vi "DAQNavi Write (Analog 1D Wfm NChan 1Samp).vi"(8 "error in (no error)":errorcluster, 9 "timeout":dbl=10.0, 10 "data":waveform(dbl)[](array[waveform]), 11 "task in":i32) -> (0 "error out":errorcluster, 2 "number of samples written per channel":u32, 3 "task out":i32)   [LabVIEW 2020]
uses:
  DAQNavi_LV.dll
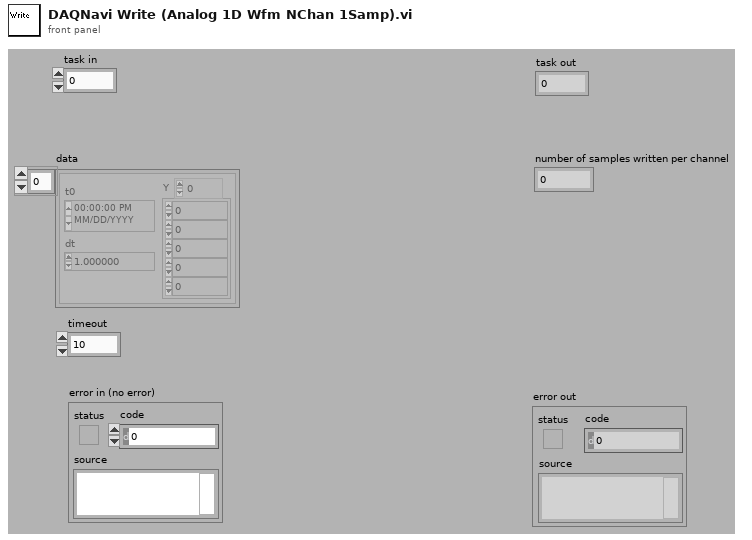
[diagram p1: front panel]
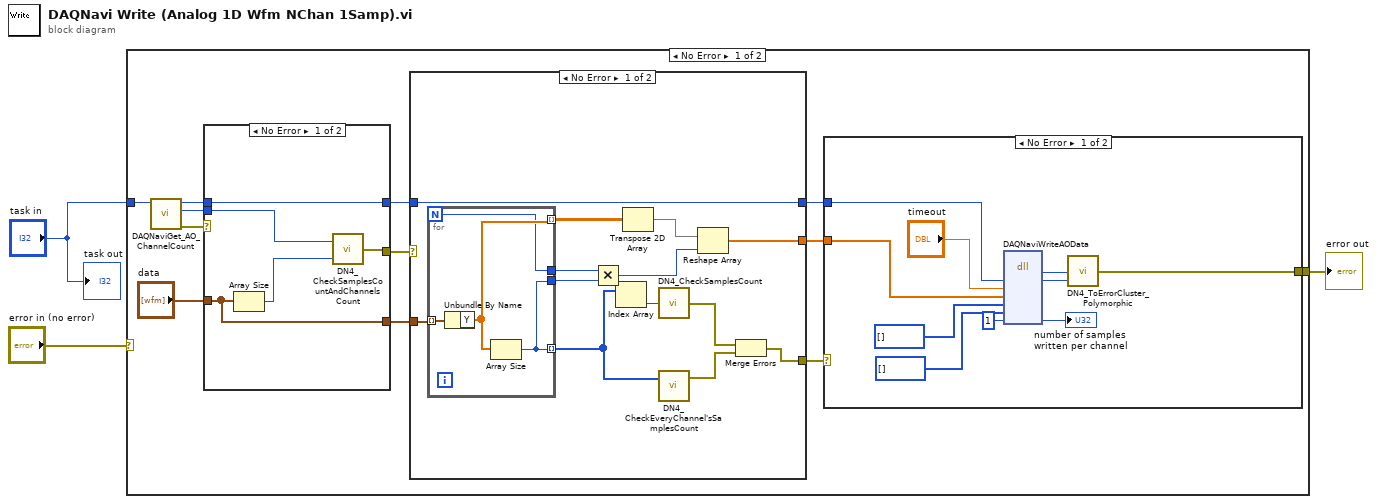
[diagram p0: block diagram]
diagram:
  n1 = case shown="No Error" "error in (no error)" {
    selector: "error in (no error)" -> [_ w54]
    tunnel: [w11 w54] -> w2
    tunnel: "task in" -> [w12 _]
    frame No Error {
      n2 = call "DAQNaviGet_AO_ChannelCount.vi"("task in"=w12) -> ("error out"=w15:errorcluster, "channel count"=w14:i32, "task out"=w13:i32)  [unwired: 1 in, 7 out]
      n3 = case shown="No Error" w15 {
        selector: w15 -> [_ w42]
        tunnel: w14 -> [w37 _]
        tunnel: [w35 w42] -> w10
        tunnel: [w39 w41] -> w7
        tunnel: w13 -> [w39 w41]
        tunnel: "data" -> [w38 w40]
        tunnel: [w38 w40] -> w9
        frame No Error {
          n4 = Array Size(array=w38) -> (size(s)=w36:i32)
          n5 = call "DN4_CheckSamplesCountAndChannelsCount.vi"("samples count"=w36, "channel count"=w37) -> ("error out"=w35:errorcluster)
        }
        frame Error {
        }
      }
      n6 = case shown="No Error" w10 {
        selector: w10 -> [_ w34]
        tunnel: w9 -> [w28 _]
        tunnel: [w23 w34] -> w8
        tunnel: [w20 w33] -> w6
        tunnel: w7 -> [w20 w33]
        tunnel: [w19 _] -> w5
        frame No Error {
          n7 = for {
            N -> [w29]
            tunnel: w28 -> [w32] mode=indexing
            tunnel: [w30] -> w27 mode=indexing
            tunnel: [w31] -> w21 mode=indexing
            tunnel: [w30] -> w18
            tunnel: [w29] -> w17
            n8 = Unbundle By Name(w32) -> ("Y"=w31:dbl[])
            n9 = Array Size(array=w31) -> (size(s)=w30:i32)
          }
          n10 = Multiply(x=w17, y=w18) -> (x*y=w16:i32)
          n11 = Index Array(array=w27) -> (element=w26:i32)  [unwired: 1 in]
          n12 = Transpose 2D Array(2D array=w21) -> (transposed array=w22:dbl[][])
          n13 = call "DN4_CheckSamplesCount.vi"("samples count"=w26) -> ("error out"=w25:errorcluster)
          n14 = call "DN4_CheckEveryChannel'sSamplesCount.vi"("samples count"=w27) -> ("error out"=w24:errorcluster)  [unwired: 1 in]
          n15 = Reshape Array(w22, w16) -> (w19:dbl[])
          n16 = Merge Errors(w25, w24) -> (w23:errorcluster)
        }
        frame Error {
        }
      }
      n17 = case shown="No Error" w8 {
        selector: w8 -> [_ w53]
        tunnel: [w52 w53] -> w11
        tunnel: w6 -> [w45 _]
        tunnel: w5 -> [w44 _]
        frame No Error {
          n18 = dll-call lib="DAQNavi_LV.dll" fn="DAQNaviWriteAOData"("taskID"=w45, "timeout"="timeout", "scaledData"=w44, "rawData16"=u16[] [], "rawData32"=u32[] [], "samples"=u32 1) -> ("return type"=w47:i32, "taskID"=w43:i32, "samples"=→"number of samples written per channel":u32)  [unwired: 5 in, 4 out]
          n19 = call "DN4_ToErrorCluster_Polymorphic.vi"("task id"=w43, "error code"=w47) -> ("error out"=w52:errorcluster)  [unwired: 3 out]
        }
        frame Error {
        }
      }
    }
    frame Error {
    }
  }
  "error out" <- w2
  "task out" <- "task in"
